vi "Write Init.vi"(1 "Network Path":string, 2 "error in":errorcluster, 3 "Int":i16, 4 "Tag Name":string) -> (0 "error out":errorcluster)   [LabVIEW 2020]
uses:
  <vilib>/ethernetip/ethernetip.llb/EthernetIP Tag Write INT.vi
  <vilib>/ethernetip/ethernetip.lvlib
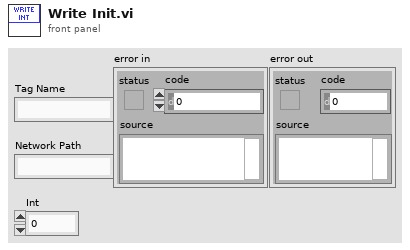
[diagram p1: front panel]
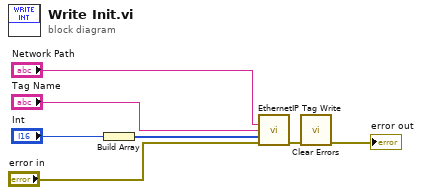
[diagram p0: block diagram]
diagram:
  n1 = Build Array("Int") -> (w5:i16[])
  n2 = call-poly <vilib>:"EthernetIP Tag Write.vi"("Network Path"="Network Path", "Tag Name"="Tag Name", "Data"=w5, "error in"="error in") -> ("error out"=w2:errorcluster)  [unwired: 10 in, 1 out]
  n3 = call <vilib>:"Clear Errors.vi"("error in (no error)"=w2) -> ("error out"=→"error out":errorcluster)  [unwired: 5 in, 1 out]
